vi "MGI Remove Array Sections.vi"(5 "child root":string, 7 "parent section":string, 8 "error in (no error)":errorcluster, 9 "New Count":i32, 10 "Old Count (-1)":i32=-1, 11 "Refnum":T1) -> (0 "error out":errorcluster, 1 "New Count out":i32, 2 "Old Count out":i32=-1, 3 "Refnum":T1)   [LabVIEW 2020]
doc: "Remove sections from an ini file when an array is shrinking. If Old Count is unwired, count will be read, parent section will be removed, and then count will be replaced. If Old Count is wired, it's assumed thatparent section handling was already performed. Child sections that are removed have names <parent>.<child root>#, where # ranges from new count to old count-1.\n\nAuthored by David A. Moore\nsupport@mooregoodideas.com\nwww.mooregoodideas.com\n\nCopyright (c) 2010, Moore Good Ideas, Inc.\n\nAll rights reserved.\n\nRedistribution and use in source and binary forms, with or without modification, are permitted provided that the following conditions are met:\n\n * Redistributions of source code must retain the above copyright notice, this list of conditions and the following disclaimer.\n * Redistributions in binary form must reproduce the above copyright notice, this list of conditions and the following disclaimer in the documentation and/or other materials provided with the distribution.\n * Neither the name of Moore Good Ideas, Inc. nor the names of its contributors may be used to endorse or promote products derived from this software without specific prior written permission.\n\nTHIS SOFTWARE IS PROVIDED BY THE COPYRIGHT HOLDERS AND CONTRIBUTORS \"AS IS\" AND ANY EXPRESS OR IMPLIED WARRANTIES, INCLUDING, BUT NOT LIMITED TO, THE IMPLIED WARRANTIES OF MERCHANTABILITY AND FITNESS FOR A PARTICULAR PURPOSE ARE DISCLAIMED. IN NO EVENT SHALL THE COPYRIGHT OWNER OR CONTRIBUTORS BE LIABLE FOR ANY DIRECT, INDIRECT, INCIDENTAL, SPECIAL, EXEMPLARY, OR CONSEQUENTIAL DAMAGES (INCLUDING, BUT NOT LIMITED TO, PROCUREMENT OF SUBSTITUTE GOODS OR SERVICES; LOSS OF USE, DATA, OR PROFITS; OR BUSINESS INTERRUPTION) HOWEVER CAUSED AND ON ANY THEORY OF LIABILITY, WHETHER IN CONTRACT, STRICT LIABILITY, OR TORT (INCLUDING NEGLIGENCE OR OTHERWISE) ARISING IN ANY WAY OUT OF THE USE OF THIS SOFTWARE, EVEN IF ADVISED OF THE POSSIBILITY OF SUCH DAMAGE.\n\nFreeware from Moore Good Ideas, www.mooregoodideas.com. Do not remove this line."
uses:
  <vilib>/Utility/config.llb/Config Data RefNum.ctl
  <vilib>/Utility/config.llb/Read Key (I32).vi
  <vilib>/Utility/config.llb/Write Key (I32).vi
  <vilib>/Utility/config.llb/NI_LVConfig.lvlib
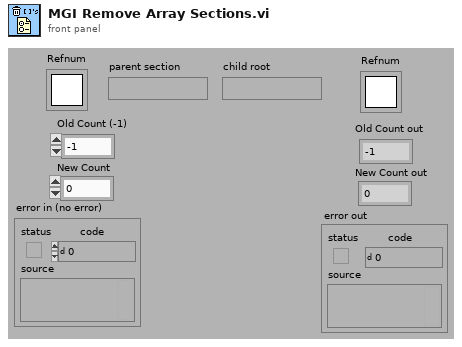
[diagram p1: front panel]
types:
  T1 = typedef "NI_LVConfig.lvlib/Config Data RefNum.ctl" = refnum<k1>
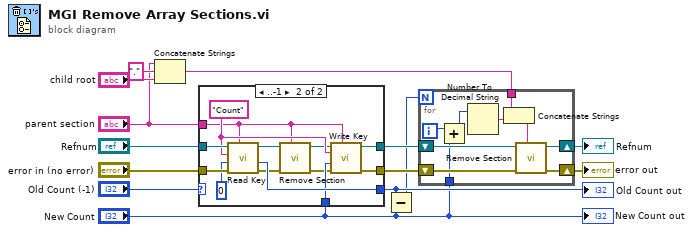
[diagram p0: block diagram]
diagram:
  n1 = Concatenate Strings("parent section", "." ("Substring"), "child root") -> (w1:string)
  n2 = case shown="..-1" "Old Count (-1)" {
    selector: "Old Count (-1)" -> [w17 _]
    tunnel: [w17 w27] -> w8
    tunnel: "New Count" -> [_ w26]
    tunnel: "error in (no error)" -> [w15 w30]
    tunnel: "Refnum" -> [w16 w29]
    tunnel: "parent section" -> [_ w18]
    tunnel: [w15 w24] -> w7
    tunnel: [w16 w23] -> w6
    frame 0.. {
    }
    frame ..-1 {
      w25 = "Count" ("key")
      n3 = call-poly <vilib>:"Read Key.vi"("section"=w18, "error in (no error)"=w30, "default value"=0, "key"=w25, "refnum"=w29) -> ("error out"=w20:errorcluster, "value"=w27:i32, "refnum out"=w19:T1)  [unwired: 3 in, 1 out]
      n4 = call <vilib>:"Remove Section.vi"("section"=w18, "error in (no error)"=w20, "refnum"=w19) -> ("error out"=w22:errorcluster, "refnum out"=w21:T1)  [unwired: 6 in, 1 out]
      n5 = call-poly <vilib>:"Write Key.vi"("section"=w18, "error in (no error)"=w22, "value"=w26, "key"=w25, "refnum"=w21) -> ("error out"=w24:errorcluster, "refnum out"=w23:T1)  [unwired: 4 in, 1 out]
    }
  }
  "Old Count out" <- w8
  n6 = Subtract(x=w8, y="New Count") -> (x-y=w5:i32)
  n7 = for {
    N: w5 -> [_]
    shift-right: [w37] -> w2
    shift-left: w7 -> [w40]
    shift-right: [w38] -> w3
    shift-left: w6 -> [w39]
    tunnel: "New Count" -> [w36]
    tunnel: w1 -> [w32]
    i -> [w35]
    n8 = Add(x=w35, y=w36) -> (x+y=w34:i32)
    n9 = Number To Decimal String(number=w34) -> (decimal integer string=w33:string)  [unwired: 1 in]
    n10 = Concatenate Strings(w32, w33) -> (w31:string)
    n11 = call <vilib>:"Remove Section.vi"("section"=w31, "error in (no error)"=w40, "refnum"=w39) -> ("error out"=w37:errorcluster, "refnum out"=w38:T1)  [unwired: 6 in, 1 out]
  }
  "error out" <- w2
  "Refnum" <- w3
  "New Count out" <- "New Count"
